vi "sensor_List.vi"() -> ()   [LabVIEW 2024]
panel:
  in  "Sensor List":cluster{"station_ID":u32, "sensor_ID":u32}[](array[cluster])
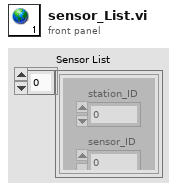
[diagram p1: front panel]
diagram:
